vi "Float Vector.vi"() -> (0 "error out":errorcluster, 3 "Passed?":bool)   [LabVIEW 2009]
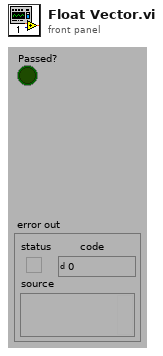
[diagram p1: front panel]
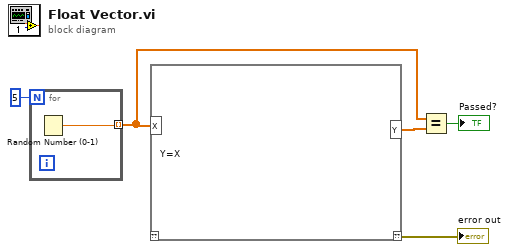
[diagram p0: block diagram]
diagram:
  n1 = for {
    N: 5 -> [_]
    tunnel: [w6] -> w2 mode=indexing
    n2 = Random Number (0-1)() -> (number: 0 to 1=w6:dbl)
  }
  n3 = script code="Y=X"("X"=w2) -> ("??"=→"error out":errorcluster, "Y"=w1:dbl[])  [unwired: 1 in]
  n4 = Equal?(x=w2, y=w1) -> (x = y?=→"Passed?":bool)
